vi "Periodic Tasks.vi"(8 "error in (no error)":errorcluster) -> ()   [LabVIEW 2011]
doc: "This VI runs in parallel to other tasks. It can contain as many user-defined periodic loops as you need. These can carry out PID or other sorts of timed response."
uses:
  <vilib>/Rock Robotics/SystemInterfaces/Utilities/FPGA_UtilitiesLED State.ctl
  <vilib>/Rock Robotics/SystemInterfaces/Utilities/FPGA_UtilitiesLED Source.ctl
  Robot Global Data.vi
panel:
  out "Autonomous Switch":dbl
  out "Already Centered":bool
  out "Encoder Direction 4":string="Backward"
  out "Encoder Alarm Status 4":string="Encoder Moving"
  in  "stop 4":bool
  out "Encoder Distance 4":dbl
  out "Encoder Rate (distance/sec) 4":dbl
  out "Encoder Direction 3":string="Backward"
  out "Encoder Alarm Status 3":string="Encoder Moving"
  in  "Reset Encoder? 3":bool
  in  "stop 3":bool
  out "Encoder Distance 3":dbl
  out "Encoder Rate (distance/sec) 3":dbl
  out "Encoder Direction 2":string="Forward"
  out "Encoder Alarm Status 2":string="Encoder Stopped"
  in  "Reset Encoder? 2":bool
  in  "stop 2":bool
  out "Encoder Distance 2":dbl=1.0
  out "Encoder Rate (distance/sec) 2":dbl
  out "Encoder Direction":string="Forward"
  out "Encoder Alarm Status":string="Encoder Stopped"
  in  "Reset Encoder?":bool
  in  "stop":bool
  out "Encoder Distance":dbl=1.0
  out "Encoder Rate (distance/sec)":dbl
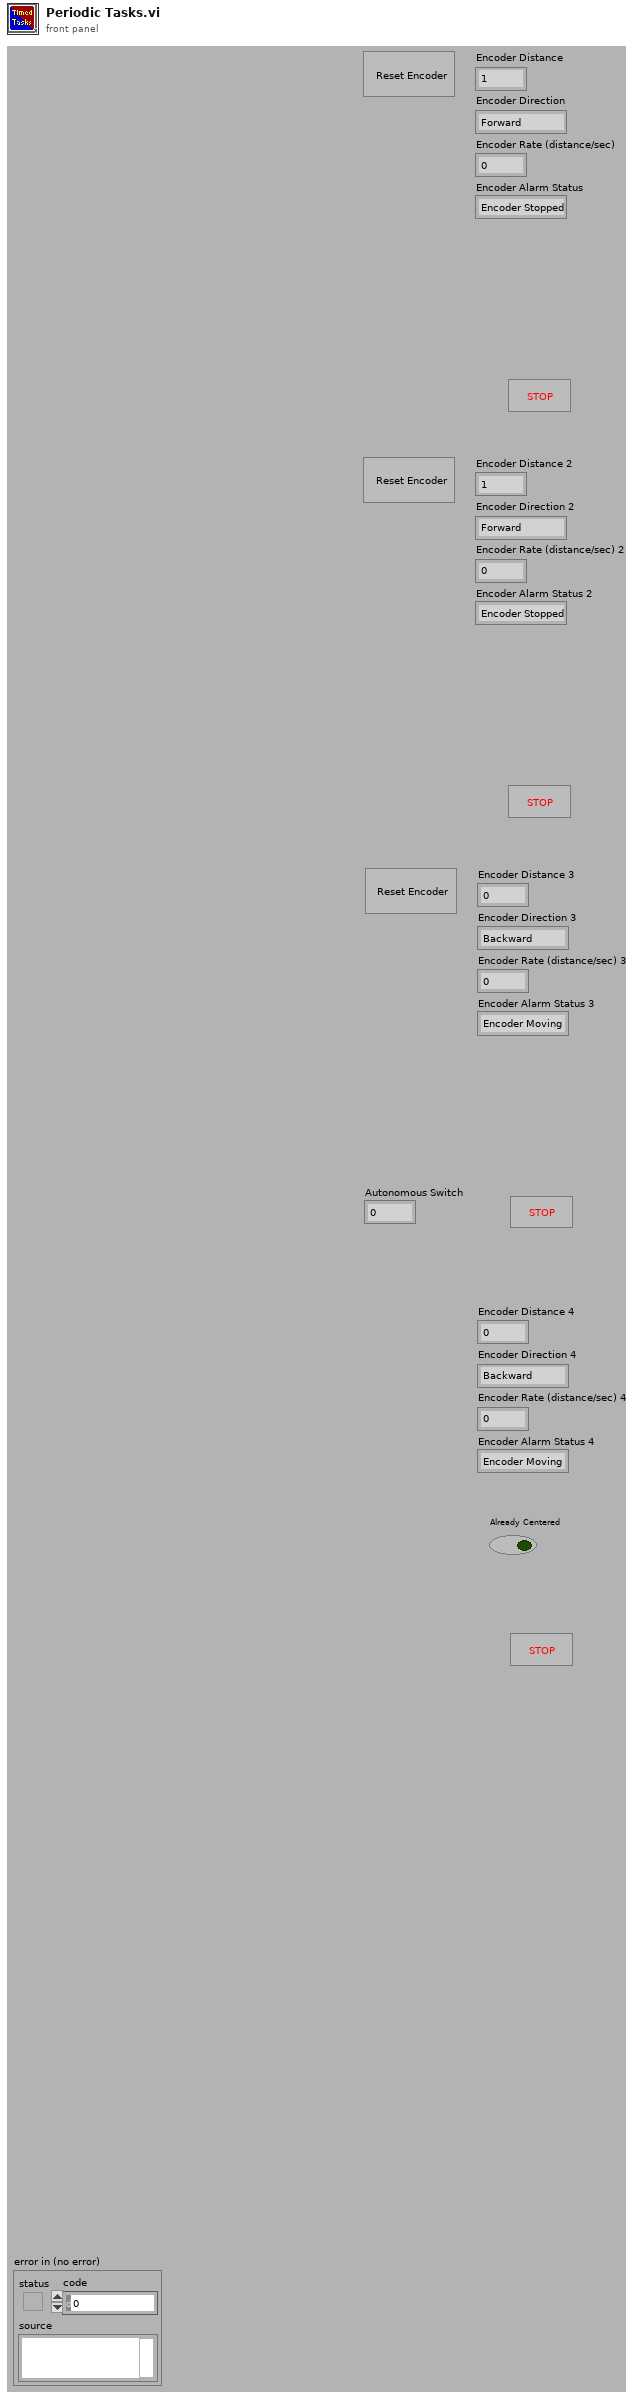
[diagram p1: front panel]
types:
  T1 = typedef "FPGA_UtilitiesLED State.ctl" = enum16{"Off", "On", "Toggle"}
  T2 = typedef "FPGA_UtilitiesLED Source.ctl" = enum16{"User LED", "FPGA LED"}
  T3 = enum16{"Shoot", "Load", "Arm", "Nothing", "Reverse", "ShootAll"}
  T4 = typedef "WPI_DigitalInputDevRef.ctl" = cluster{"DevStatus":errorcluster, "DIO Channel":T5, "Digital Module":T6}
  T5 = typedef "FPGA_DIOChannel.ctl" = enum8{"DIO 1", "DIO 2", "DIO 3", "DIO 4", "DIO 5", "DIO 6", "DIO 7", "DIO 8", "DIO 9", "DIO 10", "DIO 11", "DIO 12", "DIO 13", "DIO 14", "Invalid"}
  T6 = typedef "FPGA_TypedefDigitalModule.ctl" = enum16{"Digital Module 1", "Digital Module 2"}
  T7 = typedef "WPI_EncoderDevRef.ctl" = cluster{"DevStatus":errorcluster, "EncoderIndex":T8, "CounterIndex":T9, "DistancePerCount":dbl, "Decoding Type":T10}
  T8 = typedef "FPGA_EncoderIdx.ctl" = enum8{"Enc 0", "Enc 1", "Enc 2", "Enc 3", "Invalid"}
  T9 = typedef "FPGA_CounterCtrSystemIndex.ctl" = enum8{"Ctr 0", "Ctr 1", "Ctr 2", "Ctr 3", "Ctr 4", "Ctr 5", "Ctr 6", "Ctr 7", "Invalid"}
  T10 = typedef "WPI_EncoderType.ctl" = enum16{"1x", "2x", "4x"}
  T11 = typedef "WPI_MotorControlDeviceRef.ctl" = cluster{"DeviceStatus":errorcluster, "Type":enum16{"PWM", "CAN"}, "PWM":cluster{"Digital Module":T6, "PWM Channel":T12, "DeadBand":T13}, "CAN":cluster{"Device Number":u8, "Control Mode":T14, "Semaphore":T15, "Max Vout":dbl}, "Invert":bool, "TransformRef":T16, "InvTransformRef":T16}
  T12 = typedef "FPGA_DIOPWMChannel.ctl" = enum8{"PWM 1", "PWM 2", "PWM 3", "PWM 4", "PWM 5", "PWM 6", "PWM 7", "PWM 8", "PWM 9", "PWM 10", "Invalid"}
  T13 = typedef "WPI_PWMDeadband.ctl" = cluster{"Name":string, "maxPositivePwm":i32, "minPositivePwm":i32, "centerPwm":i32, "maxNegativePwm":i32, "minNegativePwm":i32, "angularRange":u16}
  T14 = typedef "WPI_CANJaguar_ControlMode.ctl" = enum8{"Percent VBus", "Current", "Speed", "Position", "Voltage"}
  T15 = typedef "Semaphore RefNum" = refnum<k1>
  T16 = typedef "WPI_PWMTransform_ConPane.ctl" = refnum<vi>
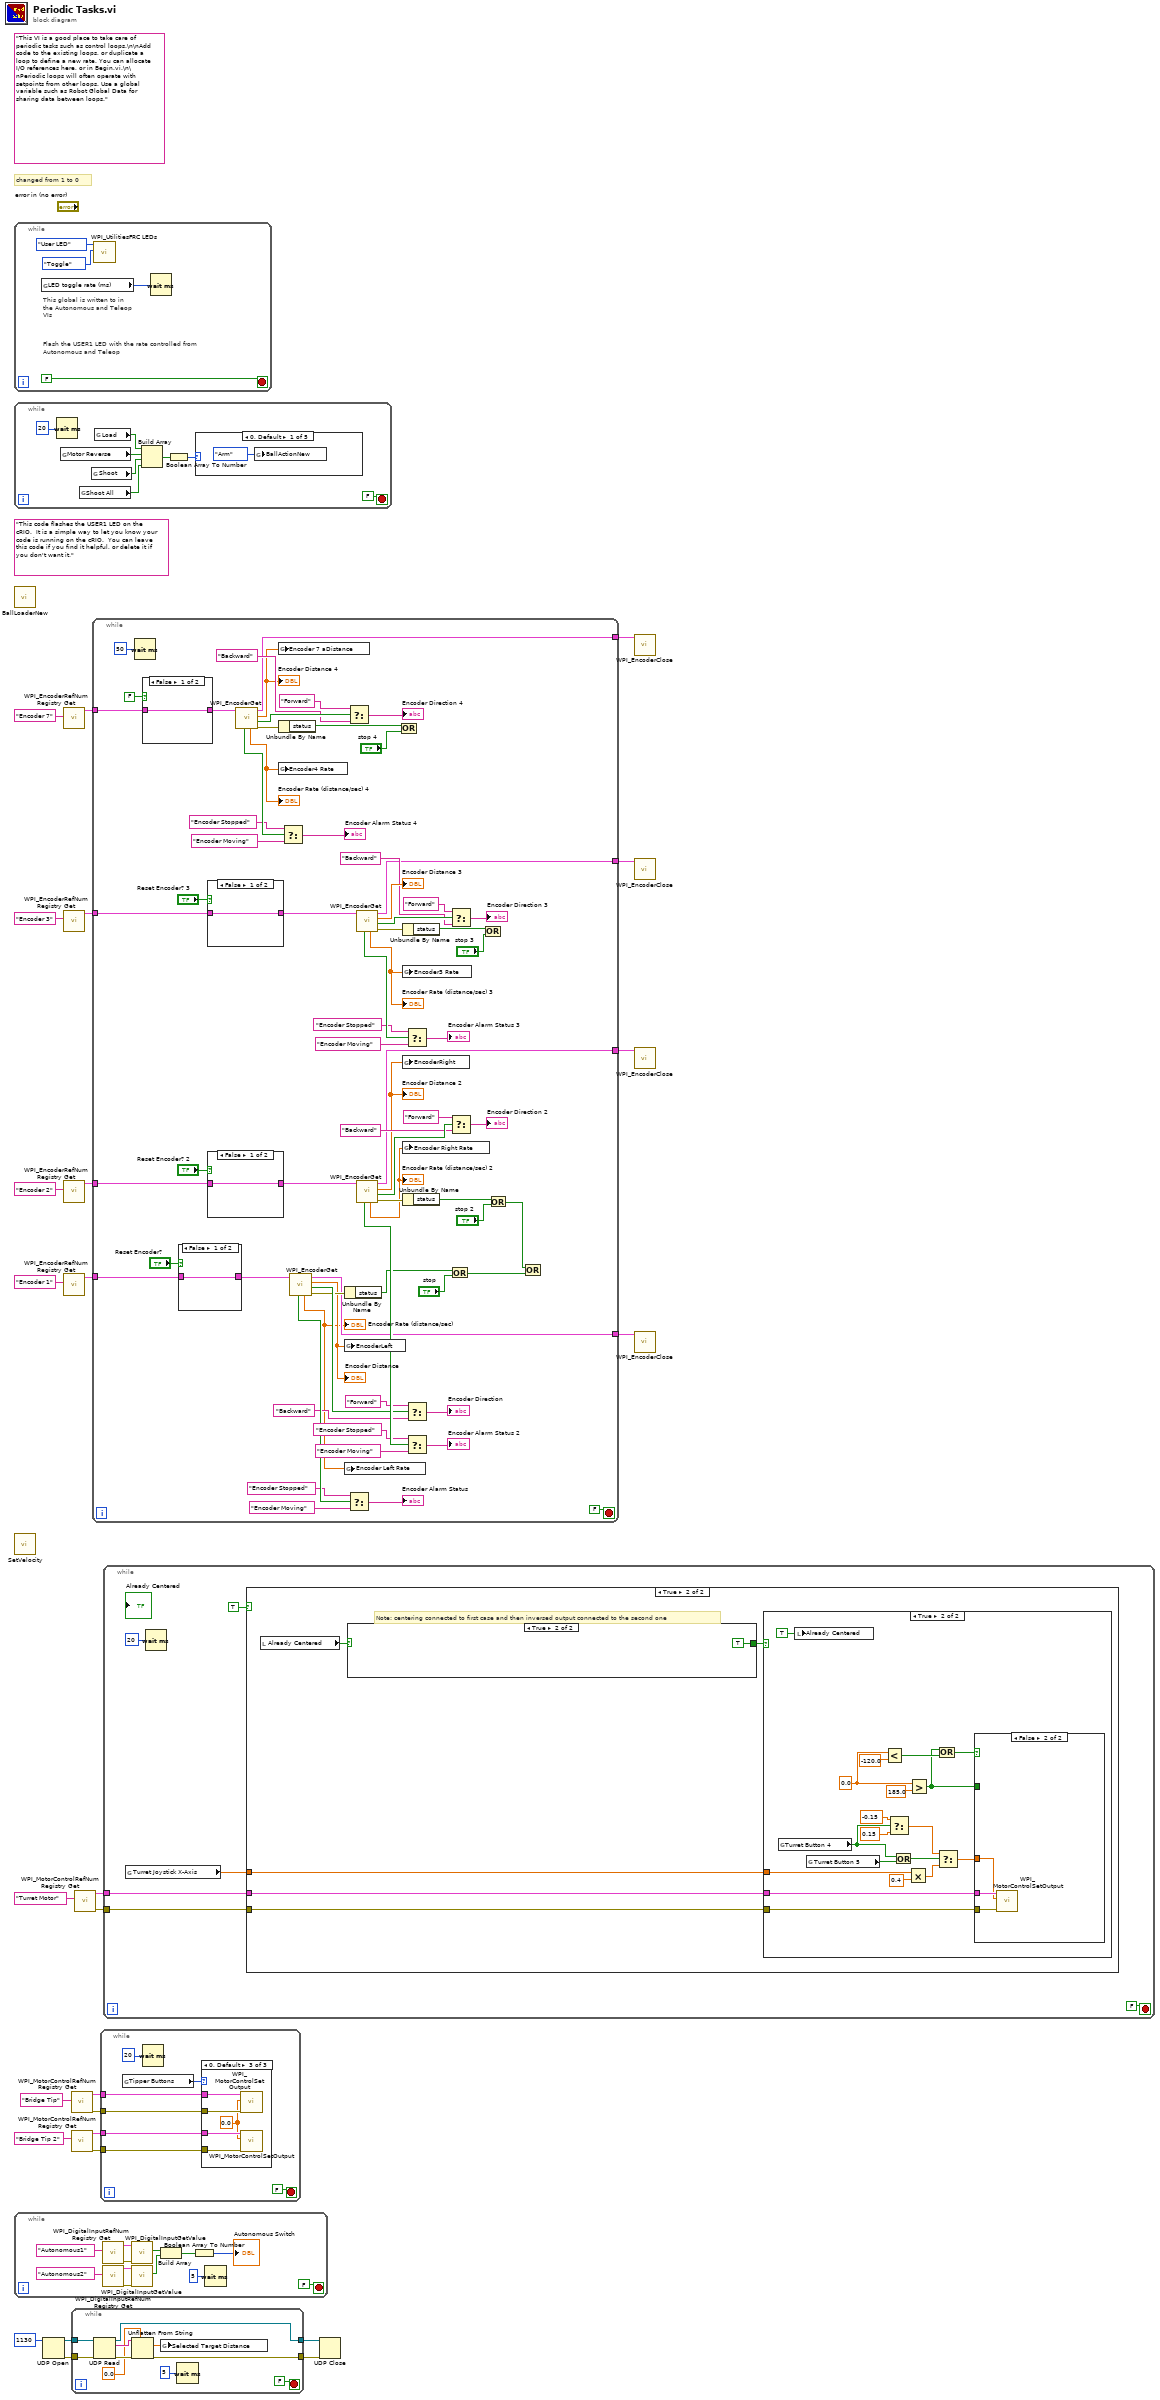
[diagram p0: block diagram]
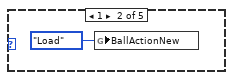
[diagram p2: hidden frame]
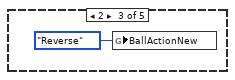
[diagram p3: hidden frame]
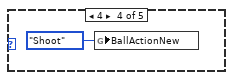
[diagram p4: hidden frame]
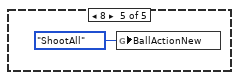
[diagram p5: hidden frame]
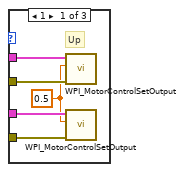
[diagram p6: hidden frame]
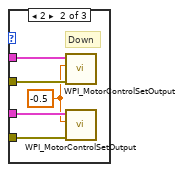
[diagram p7: hidden frame]
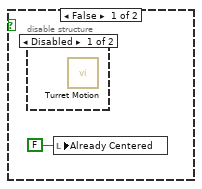
[diagram p8: hidden frame]
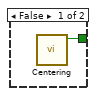
[diagram p10: hidden frame]
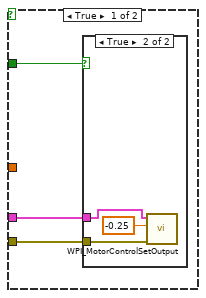
[diagram p12: hidden frame]
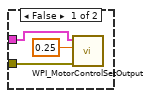
[diagram p13: hidden frame]
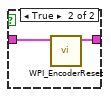
[diagram p14: hidden frame]
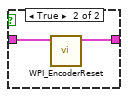
[diagram p15: hidden frame]
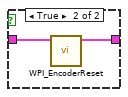
[diagram p16: hidden frame]
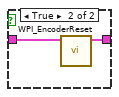
[diagram p17: hidden frame]
diagram:
  (unwired) "This VI is a good place to take care of periodic tasks such as control loops.\n\nAdd code to the existing loops, or duplicate a loop to define a new rate. You can allocate I/O references here, or in Begin.vi.\n\nPeriodic loops will often operate with setpoints from other loops. Use a global variable such as Robot Global Data for sharing data between loops."
  (unwired) "This code flashes the USER1 LED on the cRIO.  It is a simple way to let you know your code is running on the cRIO.  You can leave this code if you find it helpful, or delete it if you don't want it."
  # "changed from 1 to 0"
  n1 = while {
    stop <- FALSE stop-if-true
    # "This global is written to in the Autonomous and Teleop VIs"
    # "Flash the USER1 LED with the rate controlled from Autonomous and Teleop"
    n2 = global read "Robot Global Data.vi" "LED toggle rate (ms)"() -> (w27:u32)
    n3 = call <vilib>:"WPI_UtilitiesFRC LEDs.vi"("State"=FPGA_UtilitiesLED_State."Toggle", "LED Type"=FPGA_UtilitiesLED_Source."User LED") -> ()  [unwired: 1 in, 9 out]
    n4 = Wait (ms)(milliseconds to wait=w27) -> ()  [unwired: 1 out]
  }
  n5 = while {
    stop <- FALSE stop-if-true
    n6 = Wait (ms)(milliseconds to wait=u32 20) -> ()  [unwired: 1 out]
    n7 = global read "Robot Global Data.vi" "Motor Reverse"() -> (w36:bool)
    n8 = global read "Robot Global Data.vi" "Shoot All"() -> (w34:bool)
    n9 = global read "Robot Global Data.vi" "Shoot"() -> (w35:bool)
    n10 = global read "Robot Global Data.vi" "Load"() -> (w37:bool)
    n11 = Build Array(w37, w36, w35, w34) -> (w38:bool[])
    n12 = Boolean Array To Number(Boolean array=w38) -> (number=w33:u32)
    n13 = case shown="0, Default" w33 {
      frame 0, Default {
        n14 = global write "Robot Global Data.vi" "BallActionNew"(T3."Arm" ("BallActionNew")) -> ()
      }
      frame 1 {
        n15 = global write "Robot Global Data.vi" "BallActionNew"(T3."Load" ("BallActionNew")) -> ()
      }
      frame 2 {
        n16 = global write "Robot Global Data.vi" "BallActionNew"(T3."Reverse" ("BallActionNew")) -> ()
      }
      frame 4 {
        n17 = global write "Robot Global Data.vi" "BallActionNew"(T3."Shoot" ("BallActionNew")) -> ()
      }
      frame 8 {
        n18 = global write "Robot Global Data.vi" "BallActionNew"(T3."ShootAll" ("BallActionNew")) -> ()
      }
    }
  }
  n19 = call "BallLoaderNew.vi"() -> ()  [unwired: 12 in]
  n20 = call "SetVelocity.vi"() -> ()  [unwired: 12 in]
  n21 = while {
    stop <- FALSE stop-if-true
    n22 = call <vilib>:"WPI_DigitalInputRefNum Registry Get.vi"("refnum name"="Autonomous1") -> ("error out"=w53:errorcluster, "DigitalInputDevRef"=w52:T4)  [unwired: 9 in]
    n23 = call <vilib>:"WPI_DigitalInputRefNum Registry Get.vi"("refnum name"="Autonomous2") -> ("error out"=w50:errorcluster, "DigitalInputDevRef"=w51:T4)  [unwired: 9 in]
    n24 = call <vilib>:"WPI_DigitalInputGetValue.vi"("error in (no error)"=w53, "DigitalInputDevRef"=w52) -> ("Value"=w54:bool)  [unwired: 7 in, 2 out]
    n25 = call <vilib>:"WPI_DigitalInputGetValue.vi"("error in (no error)"=w50, "DigitalInputDevRef"=w51) -> ("Value"=w55:bool)  [unwired: 7 in, 2 out]
    n26 = Build Array(w54, w55) -> (w47:bool[])
    n27 = Boolean Array To Number(Boolean array=w47) -> (number=→"Autonomous Switch":u32)
    n28 = Wait (ms)(milliseconds to wait=u32 5) -> ()  [unwired: 1 out]
  }
  n29 = UDP Open(11:u16 1130 ("port")) -> (port=w2:refnum<k16>, 0:w1:errorcluster)  [unwired: 4 in, 1 out]
  n30 = call <vilib>:"WPI_EncoderRefNum Registry Get.vi"("refnum name"="Encoder 7") -> ("EncoderDevRef"=w25:T7)  [unwired: 9 in, 1 out]
  n31 = call <vilib>:"WPI_EncoderRefNum Registry Get.vi"("refnum name"="Encoder 3") -> ("EncoderDevRef"=w22:T7)  [unwired: 9 in, 1 out]
  n32 = call <vilib>:"WPI_EncoderRefNum Registry Get.vi"("refnum name"="Encoder 2") -> ("EncoderDevRef"=w18:T7)  [unwired: 9 in, 1 out]
  n33 = call <vilib>:"WPI_EncoderRefNum Registry Get.vi"("refnum name"="Encoder 1") -> ("EncoderDevRef"=w16:T7)  [unwired: 9 in, 1 out]
  n34 = call <vilib>:"WPI_MotorControlRefNum Registry Get.vi"("refnum name"="Bridge Tip") -> ("error out"=w9:errorcluster, "MotorControlDevRef"=w10:T11)  [unwired: 9 in]
  n35 = call <vilib>:"WPI_MotorControlRefNum Registry Get.vi"("refnum name"="Bridge Tip 2") -> ("error out"=w6:errorcluster, "MotorControlDevRef"=w7:T11)  [unwired: 9 in]
  n36 = while {
    tunnel: [w64] -> w4
    tunnel: [w60] -> w3
    tunnel: w2 -> [w63]
    tunnel: w1 -> [w59]
    stop <- FALSE stop-if-true
    n37 = UDP Read(connection ID=w63, 8:w59) -> (data out=w62:string, error out=w61:errorcluster, 3:w64:refnum<k16>)  [unwired: 2 in, 2 out]
    n38 = Unflatten From String(type=0.0, binary string=w62, error in (no error)=w61) -> (value=w57:dbl, error out=w60:errorcluster)  [unwired: 2 in, 1 out]
    n39 = global write "Robot Global Data.vi" "Selected Target Distance"(w57) -> ()
    n40 = Wait (ms)(milliseconds to wait=u32 5) -> ()  [unwired: 1 out]
  }
  n41 = call <vilib>:"WPI_MotorControlRefNum Registry Get.vi"("refnum name"="Turret Motor") -> ("error out"=w12:errorcluster, "MotorControlDevRef"=w13:T11)  [unwired: 9 in]
  n42 = while {
    tunnel: w25 -> [w81]
    tunnel: [w80] -> w24
    tunnel: w22 -> [w79]
    tunnel: [w78] -> w21
    tunnel: [w77] -> w20
    tunnel: w18 -> [w76]
    tunnel: w16 -> [w75]
    tunnel: [w74] -> w15
    stop <- FALSE stop-if-true
    n43 = Wait (ms)(milliseconds to wait=u32 50) -> ()  [unwired: 1 out]
    n44 = case shown="False" FALSE {
      tunnel: w81 -> [w147 w149]
      tunnel: [w147 w148] -> w135
      frame False {
      }
      frame True {
        n45 = call <vilib>:"WPI_EncoderReset.vi"("EncoderDevRef"=w149) -> ("EncoderDevRef"=w148:T7)  [unwired: 1 in, 9 out]
      }
    }
    n46 = case shown="False" "Reset Encoder?" {
      tunnel: w75 -> [w138 w140]
      tunnel: [w138 w139] -> w94
      frame False {
      }
      frame True {
        n47 = call <vilib>:"WPI_EncoderReset.vi"("EncoderDevRef"=w140) -> ("EncoderDevRef"=w139:T7)  [unwired: 1 in, 9 out]
      }
    }
    n48 = case shown="False" "Reset Encoder? 3" {
      tunnel: w79 -> [w144 w146]
      tunnel: [w144 w145] -> w122
      frame False {
      }
      frame True {
        n49 = call <vilib>:"WPI_EncoderReset.vi"("EncoderDevRef"=w146) -> ("EncoderDevRef"=w145:T7)  [unwired: 1 in, 9 out]
      }
    }
    n50 = case shown="False" "Reset Encoder? 2" {
      tunnel: w76 -> [w141 w143]
      tunnel: [w141 w142] -> w108
      frame False {
      }
      frame True {
        n51 = call <vilib>:"WPI_EncoderReset.vi"("EncoderDevRef"=w143) -> ("EncoderDevRef"=w142:T7)  [unwired: 1 in, 9 out]
      }
    }
    n52 = call <vilib>:"WPI_EncoderGet.vi"("EncoderDevRef"=w135) -> ("error out"=w132:errorcluster, "Direction"=w134:bool, "Distance"=w73:dbl, "EncoderDevRef"=w80:T7, "Rate"=w125:dbl, "Stopped"=w133:bool)  [unwired: 1 in, 4 out]
    "Encoder Distance 4" <- w73
    "Encoder Rate (distance/sec) 4" <- w125
    n53 = global write "Robot Global Data.vi" "Encoder 7 aDistance"(w73) -> ()
    n54 = Unbundle By Name(w132) -> ("status"=w130:bool)
    n55 = global write "Robot Global Data.vi" "Encoder4 Rate"(w125) -> ()
    n56 = Select(t="Encoder Stopped", s=w133, f="Encoder Moving") -> (s? t:f=→"Encoder Alarm Status 4":string)
    n57 = call <vilib>:"WPI_EncoderGet.vi"("EncoderDevRef"=w94) -> ("error out"=w90:errorcluster, "Direction"=w93:bool, "Distance"=w70:dbl, "EncoderDevRef"=w74:T7, "Rate"=w67:dbl, "Stopped"=w92:bool)  [unwired: 1 in, 4 out]
    "Encoder Distance" <- w70
    "Encoder Rate (distance/sec)" <- w67
    n58 = Unbundle By Name(w90) -> ("status"=w88:bool)
    n59 = global write "Robot Global Data.vi" "EncoderLeft"(w70) -> ()
    n60 = global write "Robot Global Data.vi" "Encoder Left Rate"(w67) -> ()
    n61 = Select(t="Forward", s=w134, f="Backward") -> (s? t:f=→"Encoder Direction 4":string)
    n62 = Select(t="Encoder Stopped", s=w92, f="Encoder Moving") -> (s? t:f=→"Encoder Alarm Status":string)
    n63 = call <vilib>:"WPI_EncoderGet.vi"("EncoderDevRef"=w122) -> ("error out"=w117:errorcluster, "Direction"=w121:bool, "Distance"=→"Encoder Distance 3":dbl, "EncoderDevRef"=w78:T7, "Rate"=w68:dbl, "Stopped"=w120:bool)  [unwired: 1 in, 4 out]
    "Encoder Rate (distance/sec) 3" <- w68
    n64 = call <vilib>:"WPI_EncoderGet.vi"("EncoderDevRef"=w108) -> ("error out"=w104:errorcluster, "Direction"=w107:bool, "Distance"=w69:dbl, "EncoderDevRef"=w77:T7, "Rate"=w66:dbl, "Stopped"=w106:bool)  [unwired: 1 in, 4 out]
    "Encoder Distance 2" <- w69
    "Encoder Rate (distance/sec) 2" <- w66
    n65 = Or(x=w130, y="stop 4") -> ()  [unwired: 1 out]
    n66 = Unbundle By Name(w117) -> ("status"=w115:bool)
    n67 = global write "Robot Global Data.vi" "Encoder3 Rate"(w68) -> ()
    n68 = global write "Robot Global Data.vi" "EncoderRight"(w69) -> ()
    n69 = global write "Robot Global Data.vi" "Encoder Right Rate"(w66) -> ()
    n70 = Unbundle By Name(w104) -> ("status"=w102:bool)
    n71 = Select(t="Encoder Stopped", s=w120, f="Encoder Moving") -> (s? t:f=→"Encoder Alarm Status 3":string)
    n72 = Select(t="Forward", s=w93, f="Backward") -> (s? t:f=→"Encoder Direction":string)
    n73 = Select(t="Encoder Stopped", s=w106, f="Encoder Moving") -> (s? t:f=→"Encoder Alarm Status 2":string)
    n74 = Or(x=w88, y="stop") -> (x .or. y?=w82:bool)
    n75 = Select(t="Forward", s=w121, f="Backward") -> (s? t:f=→"Encoder Direction 3":string)
    n76 = Select(t="Forward", s=w107, f="Backward") -> (s? t:f=→"Encoder Direction 2":string)
    n77 = Or(x=w115, y="stop 3") -> ()  [unwired: 1 out]
    n78 = Or(x=w102, y="stop 2") -> (x .or. y?=w83:bool)
    n79 = Or(x=w83, y=w82) -> ()  [unwired: 1 out]
  }
  n80 = while {
    tunnel: w10 -> [w153]
    tunnel: w9 -> [w152]
    tunnel: w7 -> [w151]
    tunnel: w6 -> [w150]
    stop <- FALSE stop-if-true
    n81 = global read "Robot Global Data.vi" "Tipper Buttons"() -> (w156:i32)
    n82 = Wait (ms)(milliseconds to wait=u32 20) -> ()  [unwired: 1 out]
    n83 = case shown="0, Default" w156 {
      tunnel: w153 -> [w161 w166 w171]
      tunnel: w152 -> [w160 w165 w170]
      tunnel: w151 -> [w158 w164 w169]
      tunnel: w150 -> [w159 w163 w168]
      frame 1 {
        w157 = 0.5 ("Output")
        # "Up"
        n84 = call <vilib>:"WPI_MotorControlSetOutput.vi"("error in (no error)"=w160, "Output"=w157, "MotorControlDevRef"=w161) -> ()  [unwired: 7 in, 2 out]
        n85 = call <vilib>:"WPI_MotorControlSetOutput.vi"("error in (no error)"=w159, "Output"=w157, "MotorControlDevRef"=w158) -> ()  [unwired: 7 in, 2 out]
      }
      frame 2 {
        w162 = -0.5 ("Output")
        # "Down"
        n86 = call <vilib>:"WPI_MotorControlSetOutput.vi"("error in (no error)"=w165, "Output"=w162, "MotorControlDevRef"=w166) -> ()  [unwired: 7 in, 2 out]
        n87 = call <vilib>:"WPI_MotorControlSetOutput.vi"("error in (no error)"=w163, "Output"=w162, "MotorControlDevRef"=w164) -> ()  [unwired: 7 in, 2 out]
      }
      frame 0, Default {
        w167 = 0.0 ("Output")
        n88 = call <vilib>:"WPI_MotorControlSetOutput.vi"("error in (no error)"=w170, "Output"=w167, "MotorControlDevRef"=w171) -> ()  [unwired: 7 in, 2 out]
        n89 = call <vilib>:"WPI_MotorControlSetOutput.vi"("error in (no error)"=w168, "Output"=w167, "MotorControlDevRef"=w169) -> ()  [unwired: 7 in, 2 out]
      }
    }
  }
  n90 = while {
    tunnel: w13 -> [w174]
    tunnel: w12 -> [w173]
    stop <- FALSE stop-if-true
    n91 = global read "Robot Global Data.vi" "Turret Joystick X-Axis"() -> (w177:dbl)
    n92 = Wait (ms)(milliseconds to wait=u32 20) -> ()  [unwired: 1 out]
    n93 = case shown="True" TRUE {
      tunnel: w177 -> [_ w182]
      tunnel: w174 -> [_ w183]
      tunnel: w173 -> [_ w181]
      frame False {
        n94 = disable-structure shown="Disabled" {
          frame Disabled {
            n95 = call "Turret Motion.vi"() -> ()  [unwired: 11 in]
          }
          frame Enabled {
          }
        }
        n96 = local write "Already Centered"(FALSE) -> ()
      }
      frame True {
        # "Note: centering connected to first case and then inversed output connected to the second one"
        n97 = local read "Already Centered"() -> (w180:bool)
        n98 = case shown="True" w180 {
          tunnel: [w184 TRUE ("Ready To Move On")] -> w179
          frame False {
            n99 = call "Centering.vi"() -> ("Ready To Move On"=w184:bool)  [unwired: 11 in]
          }
          frame True {
          }
        }
        n100 = case shown="True" w179 {
          tunnel: w183 -> [_ w204]
          tunnel: w182 -> [_ w196]
          tunnel: w181 -> [_ w203]
          frame False {
          }
          frame True {
            w194 = 0.0
            n101 = global read "Robot Global Data.vi" "Turret Button 4"() -> (w189:bool)
            n102 = local write "Already Centered"(TRUE ("Already Centered")) -> ()
            n103 = global read "Robot Global Data.vi" "Turret Button 5"() -> (w191:bool)
            n104 = Less?(x=w194, y=-120.0) -> (x < y?=w200:bool)
            n105 = Select(t=-0.15, s=w189, f=0.15) -> (s? t:f=w186:dbl)
            n106 = Or(x=w189, y=w191) -> (x .or. y?=w190:bool)
            n107 = Multiply(x=w196, y=0.4) -> (x*y=w192:dbl)
            n108 = Greater?(x=w194, y=185.0) -> (0:w199:bool)
            n109 = Or(x=w199, y=w200) -> (x .or. y?=w197:bool)
            n110 = Select(t=w186, s=w190, f=w192) -> (s? t:f=w193:dbl)
            n111 = case shown="False" w197 {
              tunnel: w204 -> [w205 w216]
              tunnel: w193 -> [_ w215]
              tunnel: w203 -> [w206 w214]
              tunnel: w199 -> [w207 _]
              frame True {
                n112 = case shown="True" w207 {
                  tunnel: w206 -> [w209 w211]
                  tunnel: w205 -> [w208 w212]
                  frame False {
                    n113 = call <vilib>:"WPI_MotorControlSetOutput.vi"("error in (no error)"=w209, "Output"=0.25, "MotorControlDevRef"=w208) -> ()  [unwired: 7 in, 2 out]
                  }
                  frame True {
                    n114 = call <vilib>:"WPI_MotorControlSetOutput.vi"("error in (no error)"=w211, "Output"=-0.25, "MotorControlDevRef"=w212) -> ()  [unwired: 7 in, 2 out]
                  }
                }
              }
              frame False {
                n115 = call <vilib>:"WPI_MotorControlSetOutput.vi"("error in (no error)"=w214, "Output"=w215, "MotorControlDevRef"=w216) -> ()  [unwired: 7 in, 2 out]
              }
            }
          }
        }
      }
    }
  }
  n116 = UDP Close(connection ID=w4, 8:w3) -> ()  [unwired: 2 out]
  n117 = call <vilib>:"WPI_EncoderClose.vi"("EncoderDevRef"=w24) -> ()  [unwired: 2 in, 9 out]
  n118 = call <vilib>:"WPI_EncoderClose.vi"("EncoderDevRef"=w21) -> ()  [unwired: 2 in, 9 out]
  n119 = call <vilib>:"WPI_EncoderClose.vi"("EncoderDevRef"=w20) -> ()  [unwired: 2 in, 9 out]
  n120 = call <vilib>:"WPI_EncoderClose.vi"("EncoderDevRef"=w15) -> ()  [unwired: 2 in, 9 out]
